vi "To BananaPips.vi"(10 "Test Result":refnum<class "Test Result.lvclass">) -> (3 "Pips.TestResults":refnum<class "Pips.TestResults.lvclass">)   [LabVIEW 2021, in "Banana.Caraya.lvlib" / "Pips.TestResults.lvclass"]
uses:
  Pips.TestResults.lvclass
  <vilib>/addons/_JKI Toolkits/Caraya/classes/Test Result/Test Result.lvclass
  Pips.TestResults.lvclass/Pips.TestResults.ctl
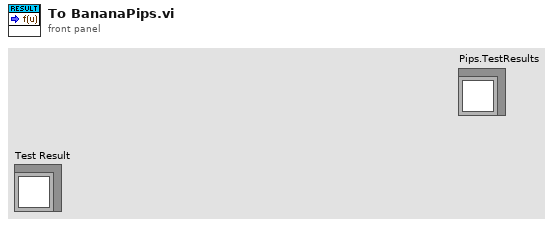
[diagram p1: front panel]
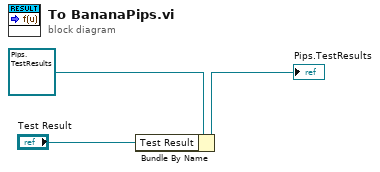
[diagram p0: block diagram]
diagram:
  n1 = Bundle By Name(cluster=refnum<class "Pips.TestResults.lvclass"> refnum ("Leaf.Properties.Assert in"), "Test Result"="Test Result") -> (→"Pips.TestResults":refnum<class "Pips.TestResults.lvclass">)
